vi "Error Processor.vi"(8 "error in (no error)":errorcluster, 11 "New uService Template in":refnum<class "Tamer.lvclass">) -> (0 "error out":errorcluster, 3 "New uService Template out":refnum<class "Tamer.lvclass">)   [LabVIEW 2020, in "TALOS.lvlib" / "Tamer.lvlib" / "Tamer.lvclass"]
doc: "Use this VI to process all the error that are solvable inside this specific uService. Whatever is not possible to process, let it leave this VI and it will be processed by the Error Manager of the Distributed System."
uses:
  Tamer.lvclass
  C:/LabVIEW Code/TALOS/talos/Father of all uServices/Father of all uServices/Father of all uServices.lvclass
  Tamer Consumer Case Selector.ctl
  Father of all uServices/Father of all uServices Messages/Consumer Msg/Consumer Msg.lvclass/Consumer Msg.ctl
  Ancestor/Ancestor/Ancestor.lvclass/Ancestor.ctl
  Father of all uServices/Father of all uServices Messages/Consumer Msg/Send Consumer.vi
  Support VIs/Substitute Error.vi
  Support VIs/Generate Error.vi
  FGV/Error Memory/Get Error Description.vi
  Support VIs/Get PC name.vi
  Ancestor/Ancestor/Read ID.vi
  Support VIs/Get Class Name.vi
  <vilib>/Utility/error.llb/Clear Errors.vi
  FGV/Error Memory/Error Memory Core.vi
  <vilib>/AdvancedString/Delimited String to 1D String Array.vi
  Support VIs/Circus Root Path.vi
  FGV/Error Memory/Error Crt Lvl checker.vi
  FGV/Error Memory/Error Memory Core.vi/40c8088d-b597-4017-91af-faa98e00292e.vi
  FGV/Error Memory/Error Memory Core.vi/d4a3ab98-063c-4e44-b43d-fbdcfe6c2be2.vi
  Father of all uServices/Father of all uServices/Father of all uServices.lvclass
  C:/LabVIEW Code/TALOS/builds/Actor Framework PPL/Actor Framework.lvlibp/1abvi3w/vi.lib/ActorFramework/Actor/Actor.lvclass
  builds/Actor Framework PPL/Actor Framework.lvlibp/1abvi3w/vi.lib/ActorFramework/Actor/Read Self Enqueuer.vi
  <userlib>/_OpenG.lib/lvdata/lvdata.llb/Get Strings from Enum__ogtk.vi
  builds/Actor Framework PPL/Actor Framework.lvlibp/1abvi3w/vi.lib/ActorFramework/Message Enqueuer/Enqueue.vi
  Support VIs/Global Memory.vi
  <vilib>/Utility/LVClass/Get LV Class Name.vi
  Support VIs/Is in Packed Library.vi
  Support VIs/TALOS Root path.vi
  Support VIs/Read CSV worksheet.vi
  Support VIs/Global Constants.vi
  <vilib>/Utility/error.llb/General Error Handler.vi
  Support VIs/Error Log.vi
  Father of all uServices/Father of all uServices Messages/Consumer Msg/Consumer Msg.lvclass
  Ancestor/Ancestor/Ancestor.lvclass
  <vilib>/Comparison/Equal/Equal Functor/Equal Functor.lvclass
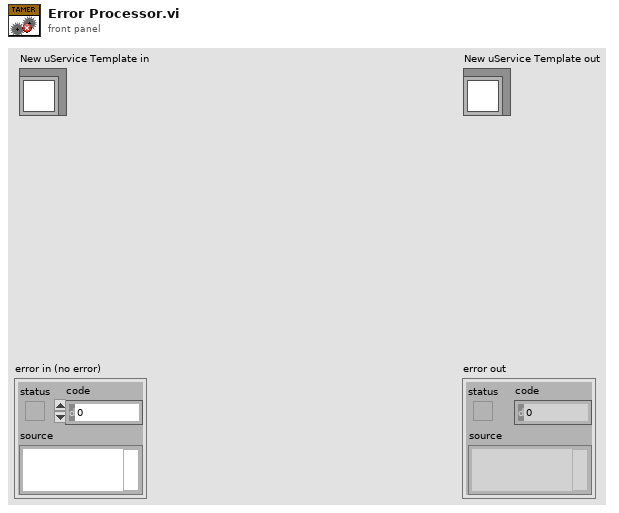
[diagram p1: front panel]
types:
  T1 = typedef "TALOS.lvlib/Tamer.lvlib/Tamer.lvclass/Tamer Consumer Case Selector.ctl" = enum16{"New schedule", "Initiate RUN", "Parse Schedules", "Script Checker", "Banana after Quality Check", "Update Crit Lvl", "Propagate Banana", "Reply from Guardian", "Reply from uService", "Timeout of RUN", "uService Replies Check", "Update from Monkey", "Monkey Died", "Reschedule", "Rerun", "Stop DAQ", "Stop Schedule", "Skip Run", "Kill Process", "Update GV"}
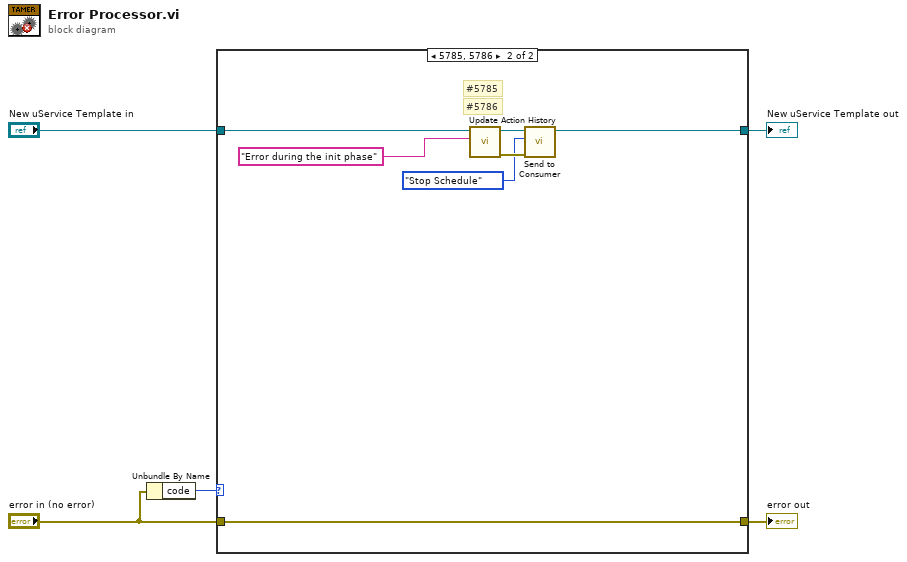
[diagram p0: block diagram]
diagram:
  n1 = Unbundle By Name("error in (no error)") -> ("code"=w2:i32)
  n2 = case shown="5785, 5786" w2 {
    tunnel: "New uService Template in" -> [w7 w10]
    tunnel: [w7 w12] -> w4
    tunnel: "error in (no error)" -> [w6 w11]
    tunnel: [w6 w11] -> w1
    frame Default {
      # "Keep the Default case as is, and generate a new case for each error  you want to process (and, hopefully, solve). All the error not managed buy this VI will be automatically handled by the Guardian and the Error Manager of the Distributed System."
    }
    frame 5785, 5786 {
      # "#5786"
      # "#5785"
      n3 = call-dynamic "Update Action History.vi"("Action"="Error during the init phase", "Tamer in"=w10) -> ("error out"=w14:errorcluster, "Tamer out"=w9:refnum<class "Tamer.lvclass">)  [unwired: 8 in]
      n4 = call "Send to Consumer.vi"("error in (no error)"=w14, "Case ID"=Tamer_Consumer_Case_Selector."Stop Schedule" ("Monkey Consumer Case Selector"), "uService Template in"=w9) -> ("uService Template out"=w12:refnum<class "Tamer.lvclass">)  [unwired: 7 in, 1 out]
    }
  }
  "error out" <- w1
  "New uService Template out" <- w4
